vi "Write Lines.vi"(8 "error in (no error)":errorcluster, 10 "Lines":T1[](array[typedef]), 11 "FPGA Module configuration in":refnum<class "FPGA Module configuration.lvclass">) -> (0 "error out":errorcluster, 3 "FPGA Module configuration out":refnum<class "FPGA Module configuration.lvclass">)   [LabVIEW 2017, in "FPGA Module configuration.lvclass"]
uses:
  FPGA Module configuration.lvclass
  Line.ctl
  fpga channel/FPGA Channel.lvclass
  FPGA Module configuration.lvclass/FPGA Module configuration.ctl
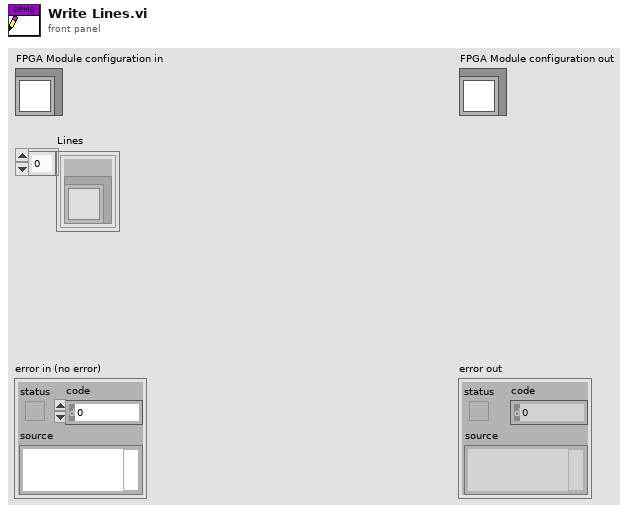
[diagram p1: front panel]
types:
  T1 = typedef "FPGA Module configuration.lvclass/Line.ctl" = cluster{"Channel":refnum<class "FPGA Channel.lvclass">}
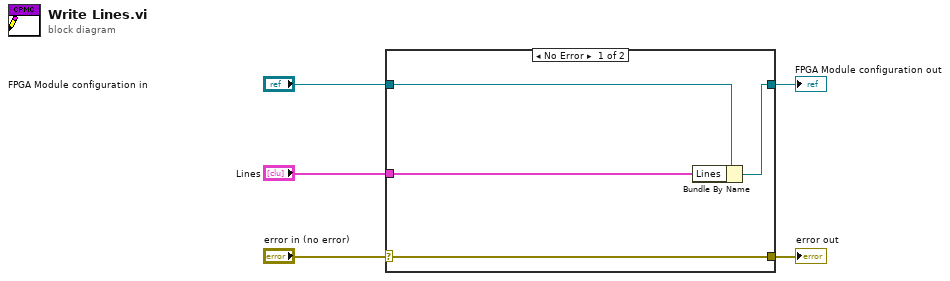
[diagram p0: block diagram]
diagram:
  n1 = case shown="No Error" "error in (no error)" {
    selector: "error in (no error)" -> [w9 w10]
    tunnel: [w9 w10] -> w4
    tunnel: [w7 w11] -> w2
    tunnel: "FPGA Module configuration in" -> [w8 w11]
    tunnel: "Lines" -> [w6 _]
    frame No Error {
      n2 = Bundle By Name(cluster=w8, "Lines"=w6) -> (w7:refnum<class "FPGA Module configuration.lvclass">)
    }
    frame Error {
    }
  }
  "error out" <- w4
  "FPGA Module configuration out" <- w2
